vi "MAP_FGV.vi"(8 "error in (no error)":errorcluster, 9 "DOs":bool[](array[boolean]), 11 "Relay_Channel_Out":T1[](array[typedef])) -> (0 "error out":errorcluster, 2 "DOs_out":bool[](array[boolean]), 3 "Relay_Channel_Out 2":T1[](array[typedef]))   [LabVIEW 2024, in "ADAM_DI.lvlib"]
uses:
  ADAM_DI.lvlib
  Relay_Enum_OUT.ctl
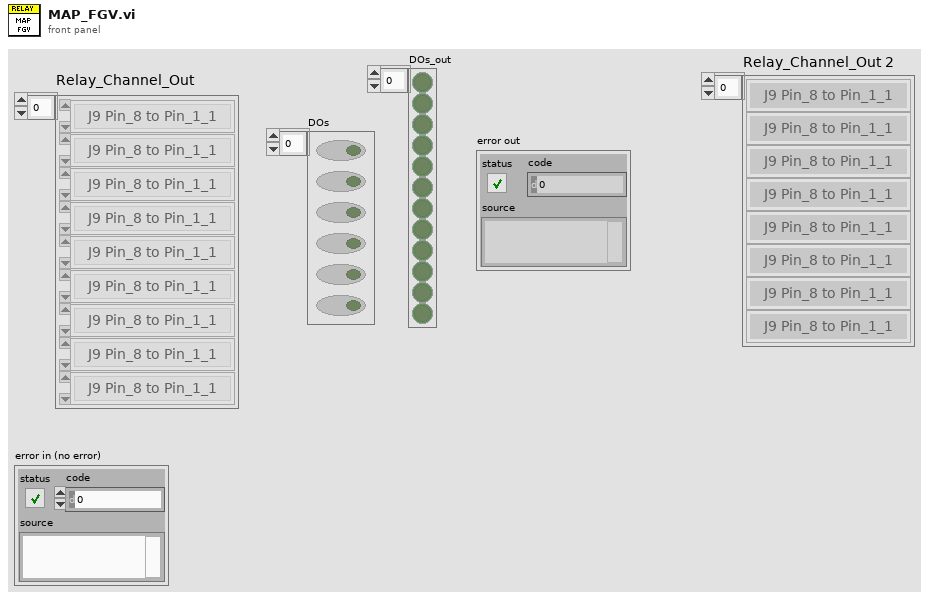
[diagram p1: front panel]
types:
  T1 = typedef "ADAM_DI.lvlib/Relay_Enum_OUT.ctl" = enum16{"J9 Pin_8 to Pin_1_1", "J9 Pin_8 to Pin_1_2", "J9 Pin_7 to Pin_1_1", "J9 Pin_7 to Pin_1_2", "J9 Pin_8 to Pin_7_1", "J9 Pin_8 to Pin_7_2", "J9 Pin_5 to Pin_1_1", "J9 Pin_5 to Pin_1_2", "J9 Pin_6 to Pin_1_1", "J9 Pin_6 to Pin_1_2", "J9 Pin_4 to Pin_1_1", "J9 Pin_4 to Pin_1_2", "J9 Pin_3 to Pin_1_1", "J9 Pin_3 to Pin_1_2", "PS(GND) to Pin1_1 J9", "PS(GND) to Pin1_2 J9", "PS(+14V) to Pin_3_1", "PS(+14V) to Pin_3_2", "PS(+12V) to Pin_4_1_ J9", "PS(+12V) to Pin_4_2_ J9", "PS(+12V) to Pin_5_1 J9", "PS(+12V) to Pin_5_2 J9", "PS(+12V) to Pin_6_1 J9", "PS(+12V) to Pin_6_2 J9", "Tower Amber", "Tower Red", "Tower Green", "Tower Buzzer", "PS(GND) to TP3_1", "PS(GND) to TP3_2", "PS(+14V) to TP19_1", "PS(+14V) to TP19_2", "PS(+12V) to TP33_1", "PS(+12V) to TP33_2", "PS(+12V) to TP38_1", "PS(+12V) to TP38_2", "PS(+12V) to TP40_1", "PS(+12V) to TP40_2", "TP19 (+14V) to TP3 (GND)_1", "TP19 (+14V) to TP3 (GND)_2", "TP1 (+14V) to TP3 (GND)_1", "TP1 (+14V) to TP3 (GND)_2", "TP2 (+5V) to TP3 (GND)_1", "TP2 (+5V) to TP3 (GND)_2", "TP6 (+14V) to TP9 (GND)_1", "TP6 (+14V) to TP9 (GND)_2", "TP7 (+3V8) to TP9 (GND)_1", "TP7 (+3V8) to TP9 (GND)_2", "TP11 (+14V) to TP13 (GND)_1", "TP11 (+14V) to TP13 (GND)_2", "TP12 (+3V) to TP13 (GND)_1", "TP12 (+3V) to TP13 (GND)_2", "TP5 (+3V3) to TP8 (GND)_1", "TP5 (+3V3) to TP8 (GND)_2", "TP48 (CAN_H) to TP3 (GND)_1", "TP48 (CAN_H) to TP3 (GND)_2", "TP41 (CAN_L) to TP3 (GND)_1", "TP41 (CAN_L) to TP3 (GND)_2", "TP48 (CAN_H) to TP41 (CAN_L)_1", "TP48 (CAN_H) to TP41 (CAN_L)_2", "TP38 (L_IND) to TP3 (GND)_1", "TP38 (L_IND) to TP3 (GND)_2", "TP40 (R_IND) to TP3 (GND)_1", "TP40 (R_IND) to TP3 (GND)_2", "TP33 (HB_CON) to TP3 (GND)_1", "TP33 (HB_CON) to TP3 (GND)_2", "TP19 (+14V) to TP34 (Q19-G)_1", "TP19 (+14V) to TP34 (Q19-G)_2", "TP55 (SW1) to TP3 (GND)_1", "TP55 (SW1) to TP3 (GND)_2", "TP56 (SW2) to TP3 (GND)_1", "TP56 (SW2) to TP3 (GND)_2", "TP66 WRT TP3 (GND)_1", "TP66 WRT TP3 (GND)_2", "TP19 WRT TP3_1", "TP19 WRT TP3_2", "TP1 WRT TP3_1", "TP1 WRT TP3_2", "TP2 WRT TP3_1", "TP2 WRT TP3_2", "TP7 WRT TP9_1", "TP7 WRT TP9_2", "TP12 WRT TP13_1", "TP12 WRT TP13_2", "TP5 WRT TP8_1", "TP5 WRT TP8_2", "TP22 WRT TP3_1", "TP22 WRT TP3_2", "TP52 WRT TP3(GND)_1", "TP52 WRT TP3(GND)_2", "TP50 WRT TP3(GND)_1", "TP50 WRT TP3(GND)_2", "TP51 WRT TP3(GND)_1", "TP51 WRT TP3(GND)_2"}
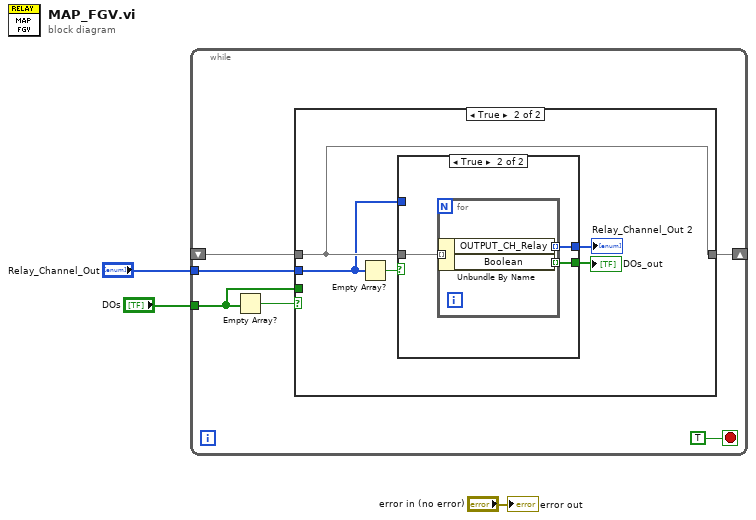
[diagram p0: block diagram]
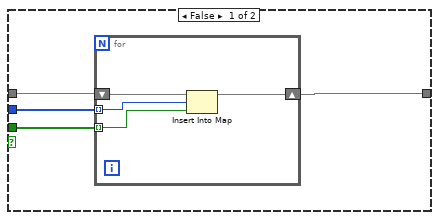
[diagram p2: hidden frame]
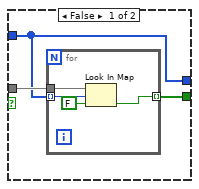
[diagram p3: hidden frame]
diagram:
  n1 = while {
    tunnel: "DOs" -> [w6]
    tunnel: "Relay_Channel_Out" -> [w7]
    shift-right: [w5] -> _
    shift-left: _ -> [w4]
    stop <- TRUE stop-if-true
    n2 = Empty Array?(array=w6) -> (empty?=w8:bool)
    n3 = case shown="True" w8 {
      tunnel: w7 -> [w13 w20]
      tunnel: w6 -> [w12 _]
      tunnel: [w11 w21] -> w5
      tunnel: w4 -> [w10 w21]
      frame False {
        n4 = for {
          tunnel: w13 -> [w17] mode=indexing
          tunnel: w12 -> [w16] mode=indexing
          shift-right: [w15] -> w11
          shift-left: w10 -> [w14]
          n5 = Insert Into Map(map in=w14, key=w17, value=w16) -> (map out=w15:map{T1, bool})  [unwired: 2 out]
        }
      }
      frame True {
        n6 = Empty Array?(array=w20) -> (empty?=w22:bool)
        n7 = case shown="True" w22 {
          tunnel: w21 -> [w25 w32]
          tunnel: [w23 w30] -> w18
          tunnel: [w24 w31] -> w19
          tunnel: w20 -> [w23 _]
          frame False {
            n8 = for {
              tunnel: w25 -> [w29]
              tunnel: [w28] -> w24 mode=indexing
              tunnel: w23 -> [w27] mode=indexing
              n9 = Look In Map(map=w29, key=w27, default value=FALSE) -> (value=w28:bool)  [unwired: 1 out]
            }
          }
          frame True {
            n10 = for {
              tunnel: w32 -> [w35] mode=indexing
              tunnel: [w34] -> w30 mode=indexing
              tunnel: [w33] -> w31 mode=indexing
              n11 = Unbundle By Name(w35) -> ("OUTPUT_CH_Relay"=w34:T1, "Boolean"=w33:bool)
            }
          }
        }
        "DOs_out" <- w19
        "Relay_Channel_Out 2" <- w18
      }
    }
  }
  "error out" <- "error in (no error)"
